vi "Set Channel Class.vi"(8 "error in":errorcluster, 11 "analog input mode in":refnum<class "Analog Input Mode.lvclass">) -> (0 "error out":errorcluster, 3 "analog input mode out":refnum<class "Analog Input Mode.lvclass">)   [LabVIEW 2020, in "Scan Engine Scripting.lvlib" / "Analog Input Mode.lvclass"]
uses:
  Analog Input Mode.lvclass
  Channel Classes/AI Channel/AI Channel.lvclass
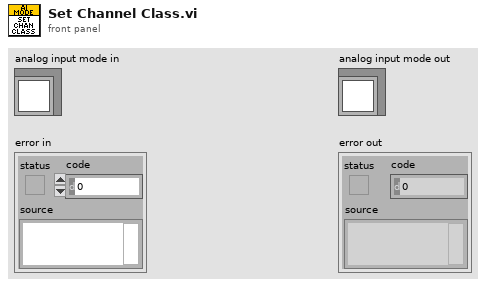
[diagram p1: front panel]
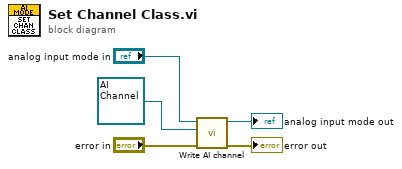
[diagram p0: block diagram]
diagram:
  n1 = call-dynamic "Write AI channel.vi"("error in"="error in", "analog input mode channel"=refnum<class "AI Channel.lvclass"> refnum ("Scan Engine Scripting.lvlib:AI Channel.lvclass"), "analog input mode in"="analog input mode in") -> ("error out"=→"error out":errorcluster, "analog input mode out"=→"analog input mode out":refnum<class "Analog Input Mode.lvclass">)  [unwired: 7 in]
